vi "Write GroupName.vi"(8 "error in":errorcluster, 10 "groupName":string, 11 "group in":refnum<class "Group.lvclass">) -> (0 "error out":errorcluster, 3 "group out":refnum<class "Group.lvclass">)   [LabVIEW 2015, in "Group.lvclass"]
uses:
  Group.lvclass
  Group.lvclass/Group.ctl
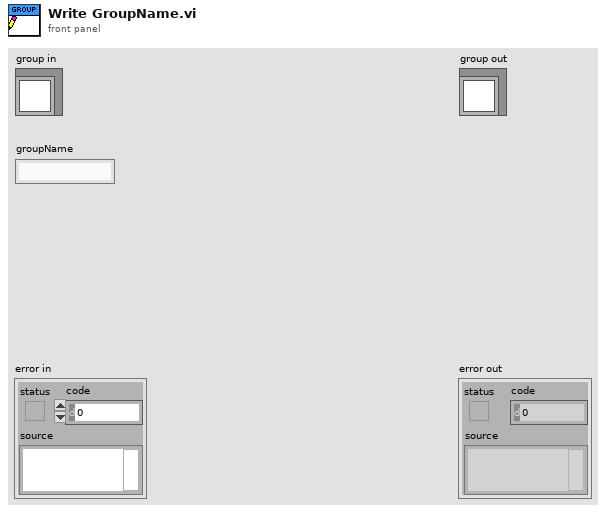
[diagram p1: front panel]
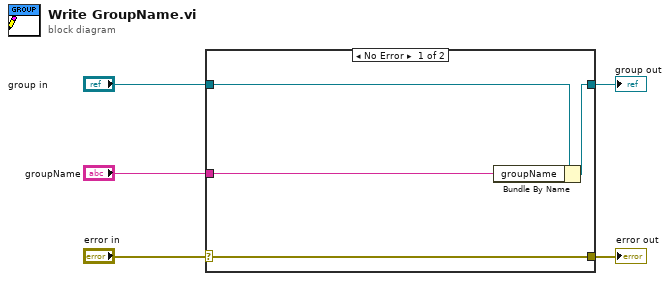
[diagram p0: block diagram]
diagram:
  n1 = case shown="No Error" "error in" {
    selector: "error in" -> [w9 w10]
    tunnel: [w9 w10] -> w4
    tunnel: [w7 w11] -> w2
    tunnel: "group in" -> [w8 w11]
    tunnel: "groupName" -> [w6 _]
    frame No Error {
      n2 = Bundle By Name(cluster=w8, "groupName"=w6) -> (w7:refnum<class "Group.lvclass">)
    }
    frame Error {
    }
  }
  "error out" <- w4
  "group out" <- w2
